vi "DEMO.vi"() -> ()   [LabVIEW 2013]
panel:
  out "Output":string
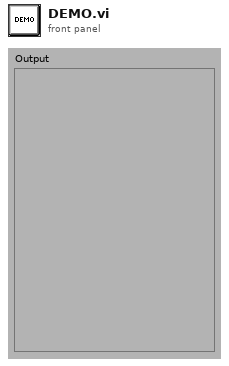
[diagram p1: front panel]
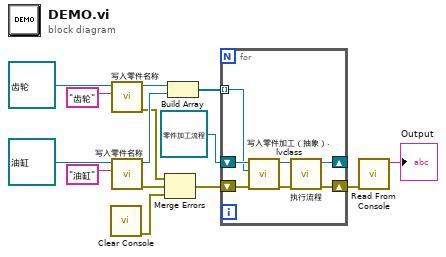
[diagram p0: block diagram]
diagram:
  n1 = call "Clear Console.vi"() -> ("error out"=w2:errorcluster)  [unwired: 11 in]
  n2 = call "写入零件名称.vi"("零件名称"="齿轮", "零件加工（抽象）输入"=refnum<class "齿轮.lvclass"> refnum ("齿轮.lvclass")) -> ("error out"=w6:errorcluster, "零件加工（抽象）输出"=w10:refnum<class "齿轮.lvclass">)  [unwired: 8 in]
  n3 = call "写入零件名称.vi"("零件名称"="油缸", "零件加工（抽象）输入"=refnum<class "油缸.lvclass"> refnum ("油缸.lvclass")) -> ("error out"=w5:errorcluster, "零件加工（抽象）输出"=w9:refnum<class "油缸.lvclass">)  [unwired: 8 in]
  n4 = Merge Errors(w6, w5, w2) -> (w4:errorcluster)
  n5 = Build Array(w10, w9) -> (w7:refnum<class "零件加工（抽象）.lvclass">[])
  n6 = for {
    shift-right: [w17] -> _
    shift-left: refnum<class "零件加工流程.lvclass"> refnum ("零件加工流程.lvclass") -> [w21]
    tunnel: w7 -> [w20] mode=indexing
    shift-right: [w16] -> w3
    shift-left: w4 -> [w15]
    n7 = call "写入零件加工（抽象）.lvclass.vi"("error in (no error)"=w15, "零件加工（抽象）.lvclass"=w20, "零件加工流程输入"=w21) -> ("error out"=w18:errorcluster, "零件加工流程输出"=w19:refnum<class "零件加工流程.lvclass">)  [unwired: 7 in]
    n8 = call "执行流程.vi"("error in (no error)"=w18, "零件加工流程 输入"=w19) -> ("error out"=w16:errorcluster, "零件加工流程 输出"=w17:refnum<class "零件加工流程.lvclass">)  [unwired: 8 in]
  }
  n9 = call "Read From Console.vi"("error in (no error)"=w3) -> ("Output"=→"Output":string)  [unwired: 9 in, 1 out]
